vi "xmlStringReadDouble.vi"(3 "error in (no error)":errorcluster, 4 "String":string) -> (0 "error out":errorcluster, 1 "Value":dbl)   [LabVIEW 2012]
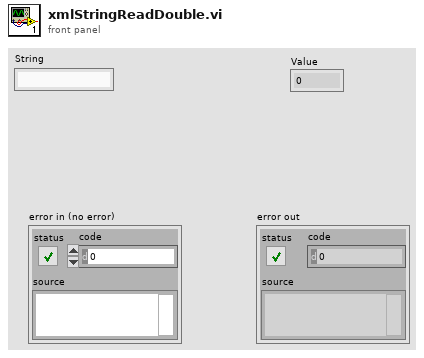
[diagram p1: front panel]
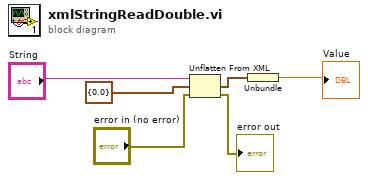
[diagram p0: block diagram]
diagram:
  n1 = Unflatten From XML(xml string="String", type=cluster{dbl} {0.0}, error in (no error)="error in (no error)") -> (value=w5:cluster{dbl}, error out=→"error out":errorcluster)
  n2 = Unbundle(w5) -> (→"Value":dbl)
